vi "repmat (dbl 2d to 2d).vi"(7 "orientation":enum16{"row", "column"}(ring), 9 "c":i32=1, 10 "r":i32=1, 11 "array in":dbl[][](array[numeric])) -> (3 "array out":dbl[][](array[numeric]))   [LabVIEW 2012, in "common.lvlib"]
uses:
  common.lvlib
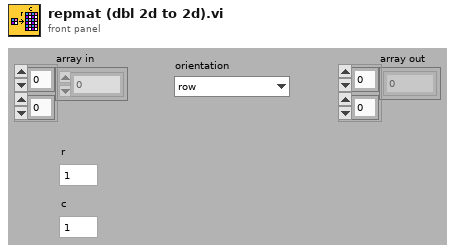
[diagram p1: front panel]
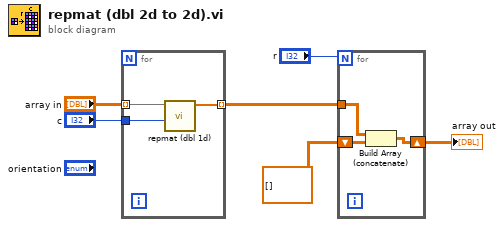
[diagram p0: block diagram]
diagram:
  n1 = for {
    tunnel: "array in" -> [w9] mode=indexing
    tunnel: "c" -> [w8]
    tunnel: [w7] -> w2 mode=indexing
    n2 = call "repmat (dbl 1d).vi"("c"=w8, "array in"=w9) -> ("array out"=w7:dbl[])  [unwired: 2 in, 7 out]
  }
  n3 = for {
    N: "r" -> [_]
    shift-right: [w10] -> w1
    shift-left: dbl[][] [] ("vector") -> [w12]
    tunnel: w2 -> [w11]
    n4 = Build Array (concatenate)(w11, w12) -> (w10:dbl[][])
  }
  "array out" <- w1
